vi "array_problem_5.vi"() -> ()   [LabVIEW 2020]
panel:
  out "result":dbl[][](array[numeric])
  in  "Array 2":dbl[][](array[numeric])
  in  "Array1":dbl[][](array[numeric])
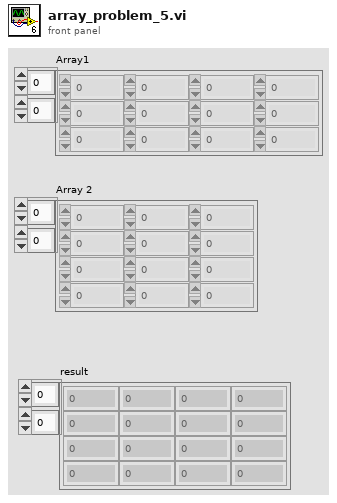
[diagram p1: front panel]
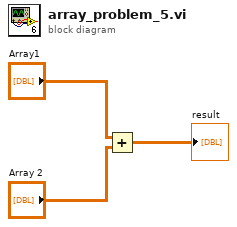
[diagram p0: block diagram]
diagram:
  n1 = Add(x="Array1", y="Array 2") -> (x+y=→"result":dbl[][])
